vi "13 - Design Pattern - Reusable Event Handlers (as a Brat VI).vi"() -> ()   [LabVIEW 2012]
panel:
  in  "Tree 3":string(tree)
  in  "Tree 2":string(tree)
  in  "Tree 1":string(tree)
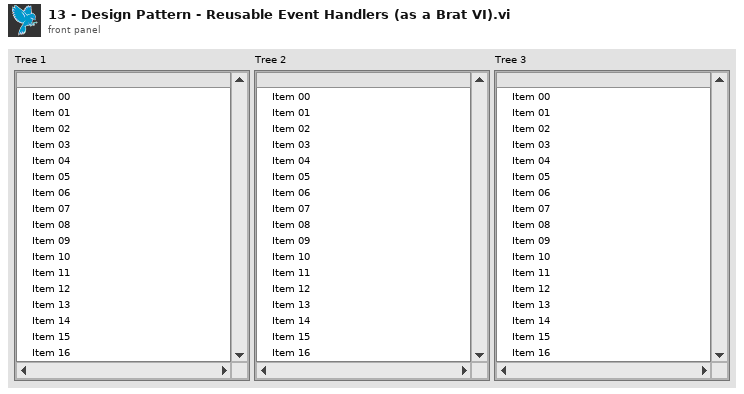
[diagram p1: front panel]
types:
  T1 = cluster{"Left Cell String":string, "Child Text":string[], "Child Tag":string, "Item Indent":i32, "Child Only?":bool, "Glyph Index":i32}
  T2 = cluster{"Enabled/Unchecked":i32, "Enabled/Checked":i32, "Disabled/Unchecked":i32, "Disabled/Checked":i32}
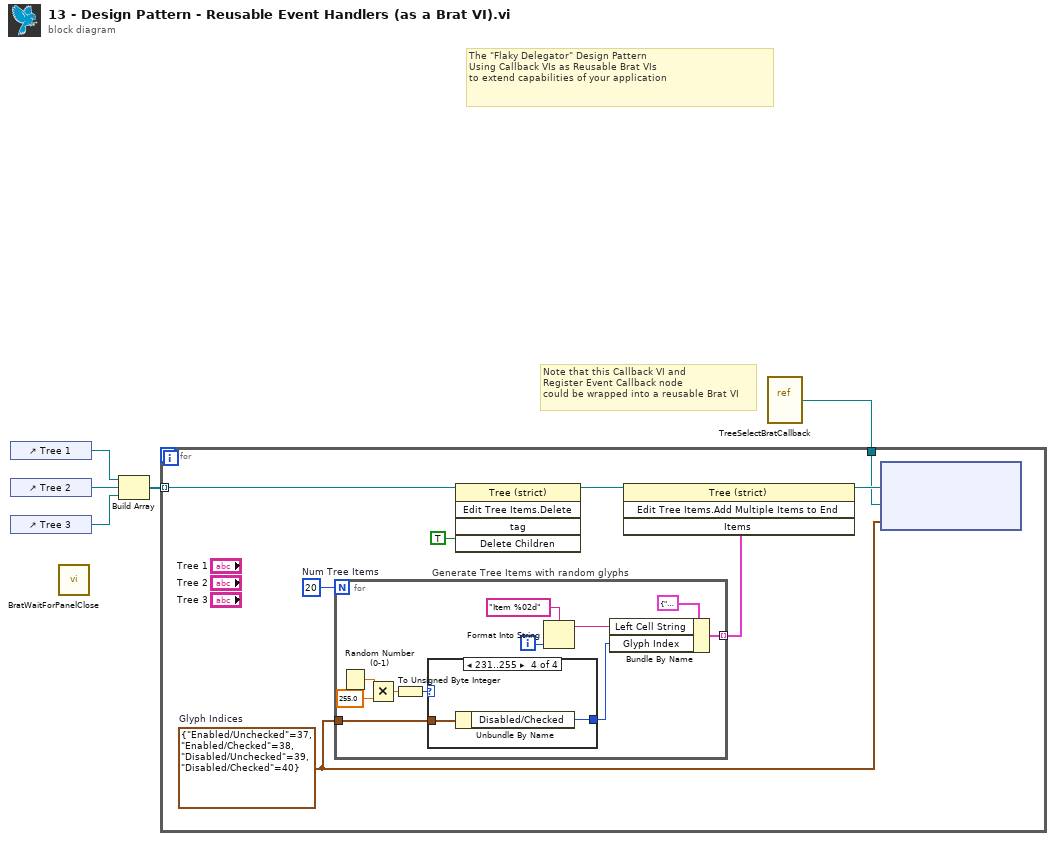
[diagram p0: block diagram]
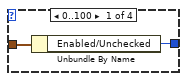
[diagram p2: hidden frame]
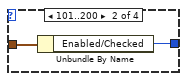
[diagram p3: hidden frame]
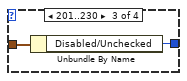
[diagram p4: hidden frame]
diagram:
  # "Note that this Callback VI and\nRegister Event Callback node\ncould be wrapped into a reusable Brat VI"
  # "The \"Flaky Delegator\" Design Pattern\nUsing Callback VIs as Reusable Brat VIs\nto extend capabilities of your application"
  n1 = control-ref of="Tree 1"() -> (w5:refnum<vi>)
  n2 = control-ref of="Tree 2"() -> (w4:refnum<vi>)
  n3 = control-ref of="Tree 3"() -> (w3:refnum<vi>)
  n4 = call "BratWaitForPanelClose.vi"() -> ()  [unwired: 12 in]
  n5 = Build Array(w5, w4, w3) -> (w2:refnum<vi>[])
  n6 = vi-ref "TreeSelectBratCallback.vi"() -> ("vi reference"=w1:refnum<vi>)
  n7 = for {
    tunnel: w2 -> [w7] mode=indexing
    tunnel: w1 -> [w6]
    w10 = 20  # Num Tree Items
    w9 = T2 {"Enabled/Unchecked"=37, "Enabled/Checked"=38, "Disabled/Unchecked"=39, "Disabled/Checked"=40}  # Glyph Indices
    n8 = for "Generate Tree Items with random glyphs" {
      N: w10 -> [_]
      tunnel: [w24] -> w13 mode=indexing
      tunnel: w9 -> [w19]
      i -> [w18]
      n9 = Random Number (0-1)() -> (number: 0 to 1=w23:dbl)
      n10 = Multiply(x=w23, y=255.0) -> (x*y=w21:dbl)
      n11 = To Unsigned Byte Integer(number=w21) -> (unsigned 8bit integer=w20:u8)
      n12 = case shown="231..255" w20 {
        tunnel: w19 -> [w26 w28 w30 w32]
        tunnel: [w25 w27 w29 w31] -> w15
        frame 0..100 {
          n13 = Unbundle By Name(w26) -> ("Enabled/Unchecked"=w25:i32)
        }
        frame 101..200 {
          n14 = Unbundle By Name(w28) -> ("Enabled/Checked"=w27:i32)
        }
        frame 201..230 {
          n15 = Unbundle By Name(w30) -> ("Disabled/Unchecked"=w29:i32)
        }
        frame 231..255 {
          n16 = Unbundle By Name(w32) -> ("Disabled/Checked"=w31:i32)
        }
      }
      n17 = Format Into String(format string="Item %02d", w18) -> (resulting string=w16:string)  [unwired: 2 in, 1 out]
      n18 = Bundle By Name(cluster=T1 {"Left Cell String"="", "Child Text"=[], "Child Tag"="", "Item Indent"=0, "Child Only?"=FALSE, "Glyph Index"=0} ("Item"), "Left Cell String"=w16, "Glyph Index"=w15) -> (w24:T1)
    }
    n19 = invoke class="Tree (strict)" method="Edit Tree Items.Delete"(reference=w7, "Delete Children"=TRUE ("Delete Children?")) -> (reference out=w11:refnum<vi>)  [unwired: 3 in, 4 out]
    n20 = invoke class="Tree (strict)" method="Edit Tree Items.Add Multiple Items to End"(reference=w11, "Items"=w13) -> (reference out=w8:refnum<vi>)  [unwired: 2 in, 3 out]
    n21 = node(w8, w6, w9) -> ()  [unwired: 2 in, 2 out]
  }
